vi "InterpolatePointsWithNumPoints.vi"(4 "x2":dbl, 6 "x1":dbl, 7 "Empty Array in":dbl[][](array[numeric]), 9 "y2":dbl, 10 "y1":dbl, 11 "Scale # points":dbl) -> (3 "Array out":dbl[][](array[numeric]))   [LabVIEW 2024]
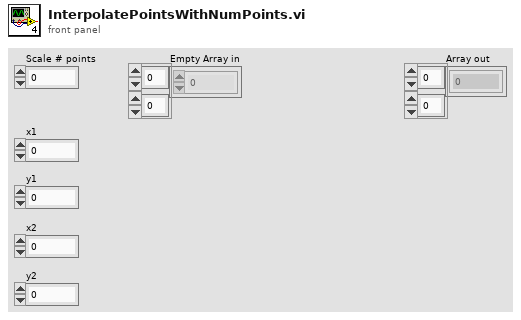
[diagram p1: front panel]
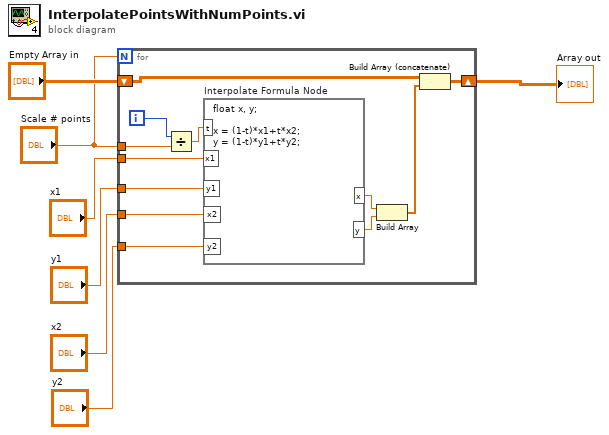
[diagram p0: block diagram]
diagram:
  n1 = for {
    N: "Scale # points" -> [_]
    tunnel: "x1" -> [w13]
    tunnel: "y1" -> [w14]
    tunnel: "y2" -> [w15]
    tunnel: "x2" -> [w16]
    tunnel: "Scale # points" -> [w17]
    shift-right: [w8] -> w6
    shift-left: "Empty Array in" -> [w9]
    i -> [w18]
    n2 = Divide(x=w18, y=w17) -> (x/y=w19:dbl)
    n3 = formula code="float x, y;\n\nx = (1-t)*x1+t*x2;\ny = (1-t)*y1+t*y2;" "Interpolate Formula Node"("x2"=w16, "y2"=w15, "t"=w19, "y1"=w14, "x1"=w13) -> ("x"=w12:dbl, "y"=w11:dbl)
    n4 = Build Array(w12, w11) -> (w10:dbl[])
    n5 = Build Array (concatenate)(w9, w10) -> (w8:dbl[][])
  }
  "Array out" <- w6
